vi "CRYMessages.vi"(0 "Setup in":T1={"No.VI"=0, "Category"="", "StepName"="", "Seq setup flattened"="", "Comment"="", "Steps config."=[], "Jump config"=[], "Start"=0.0, "Increment"=0.0, "Name"="Pa", "Unit"="Pa", "Y data"=1, "Y prefix"="", "Y dB ref"=1.0, "Y unit"="", "Repeat State Array"=[]} {"Repeat State Array"."Start" format="%#_5g"; "Y dB ref" format="%.1f"; "Y data" items=["dB", "Lin"]; "Start" format="%#_5g"}, 5 "Data in":T3[](array[typedef]) {"Z data" items=["dB", "Lin"]; "X data" items=["dB", "Lin"]; "Y data" items=["dB", "Lin"]; "Z dB ref" format="%.1f"; "Z axis" items=["Log", "Lin"]; "X dB ref" format="%.1f"; "X axis" items=["Log", "Lin"]; "Y axis" items=["Log", "Lin"]; "Y dB ref" format="%.1f"; "Curve"."z" format="%.2f"; "Curve"."y" format="%.2f"; "Curve"."x" format="%.2f"}, 7 "Results in":T4 {"Margin" format="%.2f"}, 9 "Seq Setup in":string, 11 "Step name":string, 12 "Hardware in":string, 13 "Calibration in":string) -> (3 "Types Out":string[](array[string]), 4 "Inserted Names Out":string[](array[string]), 6 "Data Out":T3[](array[typedef]) {"Z data" items=["dB", "Lin"]; "X data" items=["dB", "Lin"]; "Y data" items=["dB", "Lin"]; "Z dB ref" format="%.1f"; "Z axis" items=["Log", "Lin"]; "X dB ref" format="%.1f"; "X axis" items=["Log", "Lin"]; "Y axis" items=["Log", "Lin"]; "Y dB ref" format="%.1f"; "Curve"."z" format="%.2f"; "Curve"."y" format="%.2f"; "Curve"."x" format="%.2f"}, 8 "Results out":T4 {"Margin" format="%.2f"}, 10 "Wave out":T2[](array[typedef]) {"Y dB ref" format="%.1f"; "Y axis" items=["Log", "Lin"]; "Y data" items=["dB", "Lin"]; "X data" items=["dB", "Lin"]})   [LabVIEW 2013]
uses:
  Typedef Control/CRYData Cluster.ctl
  Typedef Control/CRYResult Cluster Array.ctl
  Typedef Control/CRYResult Cluster.ctl
  Typedef Control/CRYWaveform Cluster.ctl
  Typedef Control/CRYStep.ctl
  <vilib>/Utility/miscctls.llb/LVKeyNavTypeDef.ctl
  <vilib>/event_ctls.llb/eventvkey.ctl
  Program/CRYRef nums global.vi
  Task Sequence/CRYProject Run Control Global.vi
  CRYStepSetup/CRYStepSetup Global.vi
  CRYMainGlobal.vi
  SubVI/CRYMessage Global.vi
panel:
  out "Command":string
  in  "No":bool
  out "unit":string="(und)"
  in  "Numeric":dbl format="%#.5p"
  in  "Yes":bool
  in  "OK":bool
  out "serial line state":bool
  out "pattern":string
  out "Pattern read":T6={"0"=TRUE, "1"=TRUE, "2"=TRUE, "3"=TRUE, "4"=TRUE, "5"=TRUE, "6"=TRUE, "7"=TRUE}
  out "Write Pattern":T6={"0"=TRUE, "1"=TRUE, "2"=TRUE, "3"=TRUE, "4"=TRUE, "5"=TRUE, "6"=TRUE, "7"=TRUE}
  out "Time":u32(slide)=16203 caption="等待" scale=-1.0..1000.0
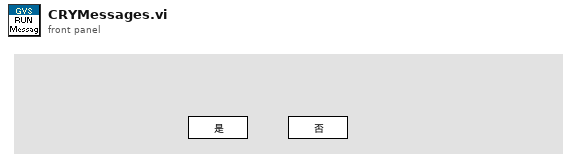
[diagram p1: front panel]
types:
  T1 = typedef "CRYStep.ctl" = cluster{"No.VI":i32, "Category":string, "StepName":string, "Seq setup flattened":string, "Comment":string, "Steps config.":bool[], "Jump config":i32[], "Start":dbl, "Increment":dbl, "Name":string, "Unit":string, "Y data":u16, "Y prefix":string, "Y dB ref":dbl, "Y unit":string, "Repeat State Array":cluster{"Start":dbl, "Increment":dbl, "Count":i32, "Num":i32}[]}
  T2 = typedef "CRYWaveform Cluster.ctl" = cluster{"Waveform":cluster{"X0":dbl, "dX":dbl, "Y":sgl[]}, "X data":u16, "Y data":u16, "Y axis":u16, "X unit":string, "Y unit":string, "Y dB ref":dbl, "display Y":bool, "display X":bool, "Overload?":bool, "Test Info":string, "Step No.":i32, "Name":string, "protected":bool, "Sqc history":string[], "Signal Channel ID":i32, "Plot Settings":cluster{"Color":u32, "Interpolation":u8, "Point Style":u8, "Line Style":u8, "Point Color":u32, "Line Width":u8, "Bar Plot Style":u8, "Fill To":i16}, "AutoProtect":bool}
  T3 = typedef "CRYData Cluster.ctl" = cluster{"Name":string, "Curve":cluster{"x":dbl, "y":dbl, "z":dbl}[], "X data":u16, "Y data":u16, "Z data":u16, "X axis":u16, "Y axis":u16, "Z axis":u16, "X unit":string, "Y unit":string, "Z unit":string, "X dB ref":dbl, "Y dB ref":dbl, "Z dB ref":dbl, "single val":bool, "protected":bool, "display X":bool, "display Y":bool, "display Z":bool, "Test Info":string, "Step No.":i32, "Plot Settings":cluster{"Color":u32, "Interpolation":u8, "Point Style":u8, "Line Style":u8, "Point Color":u32, "Line Width":u8, "Bar Plot Style":u8, "Fill To":i16}, "AutoProtect":bool}
  T4 = typedef "CRYResult Cluster Array.ctl" = T5[]
  T5 = typedef "CRYResult Cluster.ctl" = cluster{"Name":string, "Margin":dbl, "unit":string, "Verdict":bool, "Limit":string, "Max/Min":string, "protected":bool, "Step No.":i32, "Test Info":string, "AutoProtect":bool}
  T6 = cluster{"0":bool, "1":bool, "2":bool, "3":bool, "4":bool, "5":bool, "6":bool, "7":bool}
  T7 = typedef "LVKeyNavTypeDef.ctl" = cluster{"Control":bool, "Shift":bool, "Key":string}
  T8 = cluster{"Start":dbl, "Increment":dbl, "Count":i32, "Num":i32}[]
  T9 = typedef "CRYHardware.ctl" = cluster{"Name":string, "Analog I/O":u16, "Digital I/O":u16, "Channels":u8, "Dig Dev ID":u8, "N ports":u8, "Interface":u32, "Dig I/O Ports":cluster{"port #":i16, "width":i16, "direction":i32}[], "Interf settings":cluster{"Type":u16, "COM Port":u8, "Baud rate":u32, "Data bits":u32, "Parity":u16, "Stop bits":u16, "Flow control":u16, "Dev ID IEEE":u8}[], "N interfs":i32, "udev SNs":i16[], "udev enable":bool, "Channel Array":T10[], "Cal sequence":string, "SelectedIn":u16, "SelectedOut":u16, "SelectedTab":u16, "State":bool, "Help":string, "Advanced":bool, "In Audio Driver":u16, "Out Audio Driver":u16}
  T10 = typedef "CRYHardware Channel Info.ctl" = cluster{"ID":i32, "Name":string, "Digital":bool, "Input":bool, "Device Name":string, "Hardware Ch ID":u8, "Vmax (V)":dbl, "Latency (samples)":dbl, "Sampling Rate (Hz)":u32, "Bit Depth":u32, "Anti-aliasing Factor (%fs)":sgl, "DAQmx Channel":tag, "term config":i32, "Coupling":i32, "IEPE en":bool, "ASIOChannel Name":string, "Audio Driver":u16, "ASIOChannel Index":u8}
  T11 = cluster{"Type":u16, "COM Port":u8, "Baud rate":u32, "Data bits":u32, "Parity":u16, "Stop bits":u16, "Flow control":u16, "Dev ID IEEE":u8}[]
  T12 = typedef "CRYMessages Cluster.ctl" = cluster{"Name":string, "Type":u16, "Command Msg":string, "Flags":u16, "Dialog?":bool, "Numeric?":bool, "Wait?":bool, "Pause [ms]":i32, "pattern":u32, "Address":string, "Operation":i32, "bytes":i32, "Line selected":u32, "RS232 Func":u16, "Serial Ctrl lines":u16, "Interf #":u8, "GPIB func":u16, "GPIB cmd":u16, "GPIB rem en":bool, "GPIB term":i32, "Curves generated":string[], "Units":cluster{"unit":string, "dB ref":dbl, "axis":u16, "data":u16, "Common dB ref.":u16}, "Axis":u16, "Default Value":dbl, "Message Tilte":string, "Port #":i32, "Print Unit":string, "Text Format":cluster{"Size":u32, "Plain":bool, "Bold":bool, "Italic":bool, "Underline":bool, "Strikethrough":bool, "Color":u32, "Font":string}, "Help":string, "Tab Value":enum32{"Setting", "Help"}, "pattern 2":u32, "Line selected 2":u32, "H_Bits":cluster{"Bits":string[], "Invert":bool, "All":bool}[], "G_Bits":cluster{"Bits":string[], "Invert":bool, "All":bool}[]}
  T13 = cluster{"Type":u16, "COM Port":u8, "Baud rate":u32, "Data bits":u32, "Parity":u16, "Stop bits":u16, "Flow control":u16, "Dev ID IEEE":u8}
  T14 = enum32{"Invalid", "Default", "Floating", "Floating/Auto-Hide", "Modal"}
  T15 = typedef "eventvkey.ctl" = enum16{"ASCII", "Enter", "Return", "Shift", "Ctrl", "Alt", "Cmd", "Opt", "Caps", "NumLock", "Clear", "Break", "Up", "Down", "Left", "Right", "Insert", "Delete", "Home", "End", "PageUp", "PageDown", "Escape", "Help", "Pause", "ScrollLock", "F1", "F2", "F3", "F4", "F5", "F6", "F7", "F8", "F9", "F10", "F11", "F12", "F13", "F14", "F15", "F16", "F17", "F18", "F19", "F20", "F21", "F22", "F23", "F24", "Play", "VolumeUp", "VolumeDown", "Mute", "Two Byte Char"}
  T16 = enum16{"Sticks Top/Left", "Sticks Bottom/Right", "Proportional"}
  T17 = enum16{"OK", "Yes", "YesNo", "YesNoCancel", "ReplaceAppend"}
  T18 = cluster{"Size":u32, "Plain":bool, "Bold":bool, "Italic":bool, "Underline":bool, "Strikethrough":bool, "Color":u32, "Font":string}
  T19 = typedef "LVFontTypeDef.ctl" = cluster{"Font Name":string, "Size":u16, "Bold":bool, "Italic":bool, "Underline":bool, "Strikeout":bool, "Color":u32}
  T20 = typedef "LVRectTypeDef.ctl" = cluster{"Left":i16, "Top":i16, "Right":i16, "Bottom":i16}
  T21 = cluster{"unit":string, "dB ref":dbl, "axis":u16, "data":u16, "Common dB ref.":u16}
  T22 = cluster{"Numeric":dbl, "Numeric Entry":dbl, "Numeric Entry":dbl}
  T23 = cluster{"Numeric":dbl, "Numeric":dbl, "Numeric":dbl}
  T24 = cluster{"Numeric Entry":dbl, "Numeric Entry":dbl, "Numeric":dbl}
  T25 = cluster{"Numeric Entry":dbl, "Numeric Entry":dbl, "Numeric":dbl}[]
  T26 = cluster{"Bits":string[], "Invert":bool, "All":bool}[]
  T27 = cluster{"Boolean array[0]":bool, "Boolean array[1]":bool, "Boolean array[2]":bool, "Boolean array[3]":bool, "Boolean array[4]":bool, "Boolean array[5]":bool, "Boolean array[6]":bool, "Boolean array[7]":bool}
  T28 = cluster{"DIO Port Config":refnum<vi>, "DIO Port Write":refnum<vi>, "DIO Port Read":refnum<vi>}
  T29 = cluster{"COM port (1 = COM1, etc.)":i32, "VISA session (for class)":refnum<visa-resource-name>}[]
  T30 = cluster{"COM port (1 = COM1, etc.)":i32, "VISA session (for class)":refnum<visa-resource-name>}
  T31 = typedef "CRYData Cluster Array.ctl" = T3[]
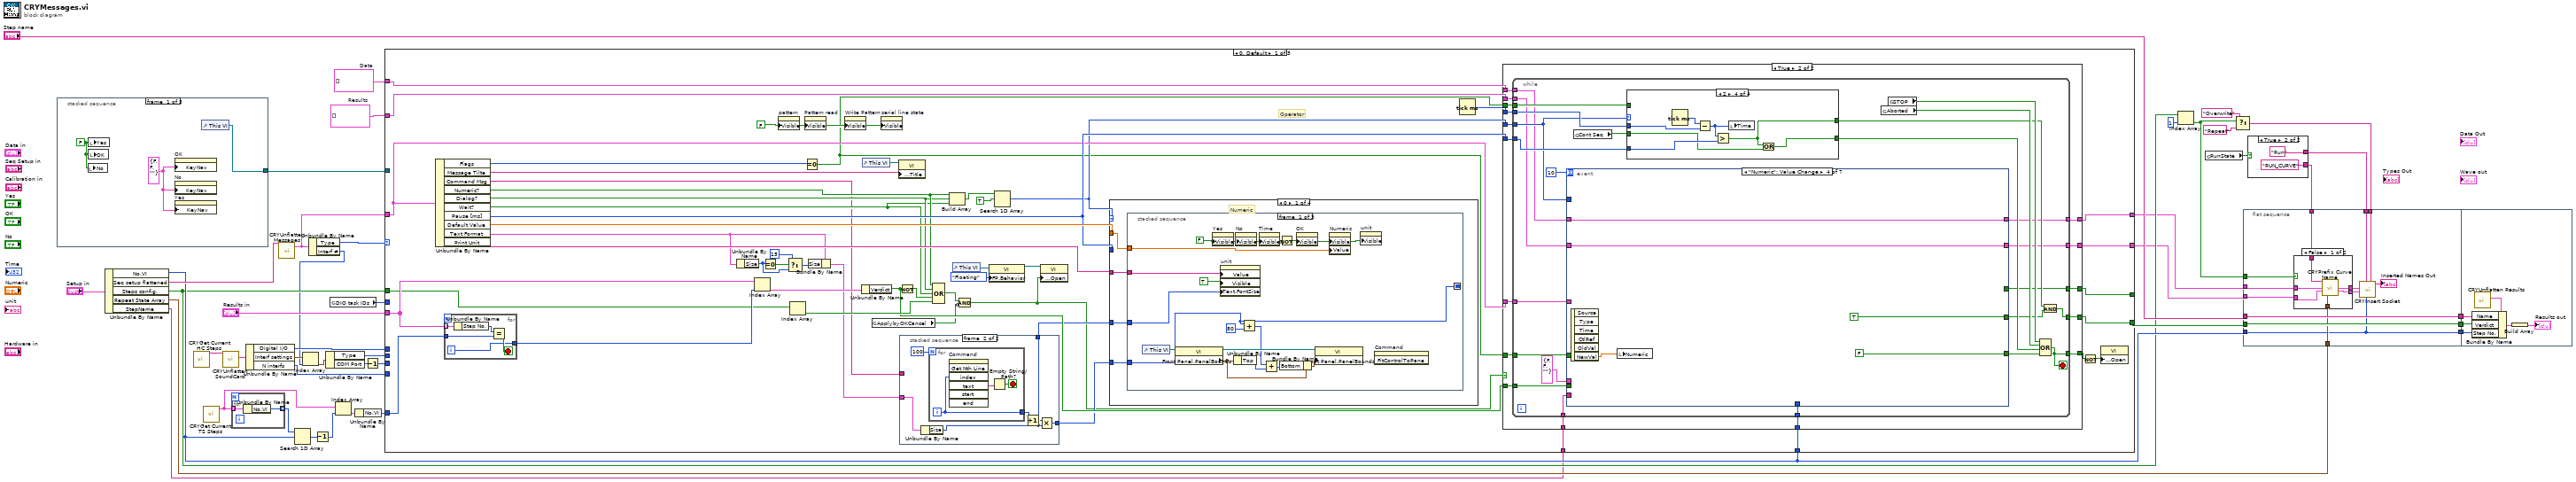
[diagram p0: block diagram]
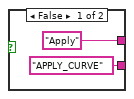
[diagram p2: hidden frame]
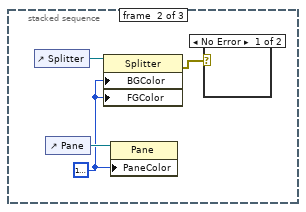
[diagram p4: hidden frame]
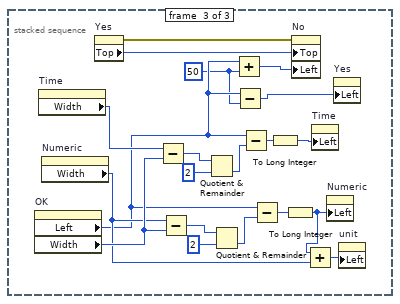
[diagram p6: hidden frame]
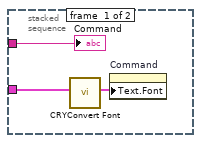
[diagram p7: hidden frame]
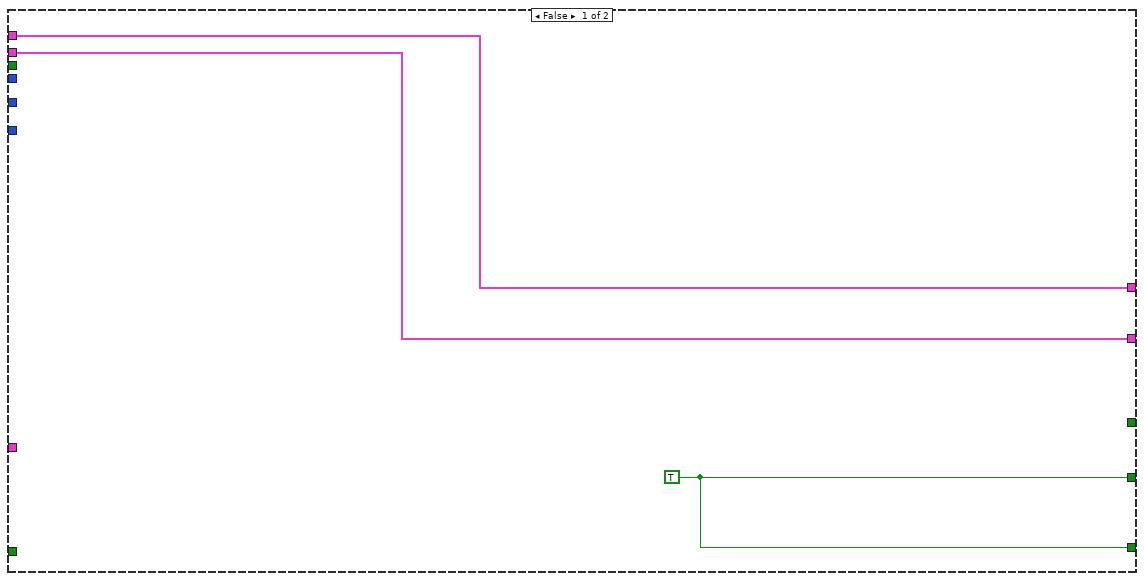
[diagram p8: hidden frame]
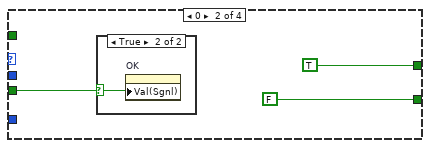
[diagram p10: hidden frame]
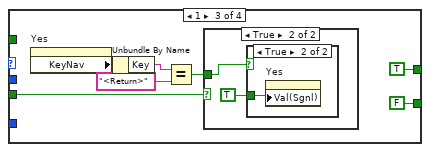
[diagram p12: hidden frame]
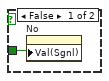
[diagram p14: hidden frame]
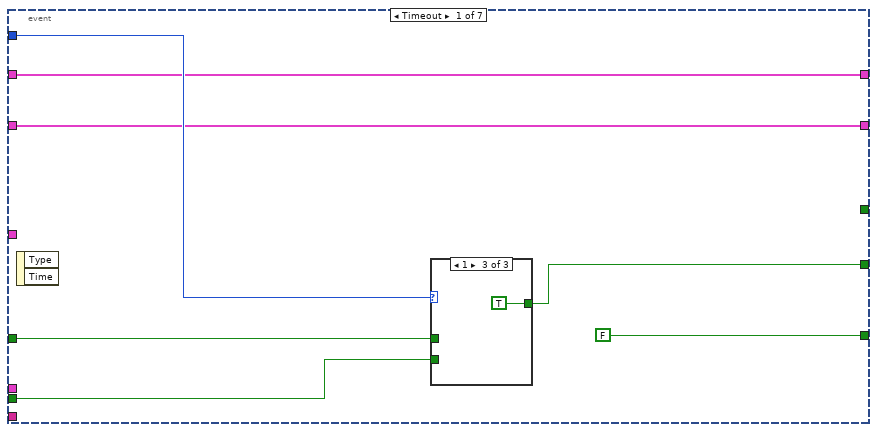
[diagram p15: hidden frame]
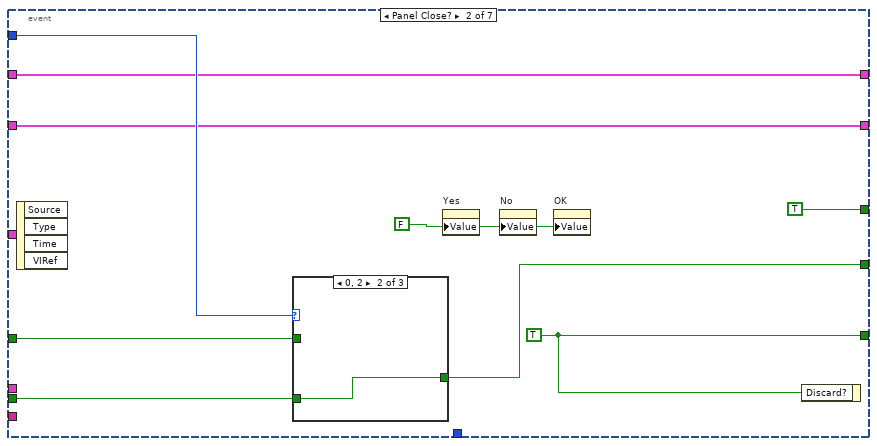
[diagram p18: hidden frame]
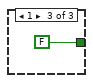
[diagram p20: hidden frame]
diagram:
  w6 = T3[] []  # Data
  w5 = T4 []  # Results
  n1 = stacked-sequence {
    tunnel: [w47 _ _] -> w29
    frame #0 {
      w45 = T7 {"Control"=FALSE, "Shift"=FALSE, "Key"=""} ("Focus Key Binding")
      w46 = FALSE ("Yes")
      n2 = local write "No"(w46) -> ()
      n3 = local write "Yes"(w46) -> ()
      n4 = local write "OK"(w46) -> ()
      n5 = property on="OK" class="Bool (strict)"("KeyNav"=w45) -> ()  [unwired: 2 in, 2 out]
      n6 = property on="No" class="Bool (strict)"("KeyNav"=w45) -> ()  [unwired: 2 in, 2 out]
      n7 = property on="Yes" class="Bool (strict)"("KeyNav"=w45) -> ()  [unwired: 2 in, 2 out]
      n8 = control-ref of="This VI"() -> (w47:refnum<vi>)
    }
    frame #1 {
      w49 = u32 16777238
      n9 = control-ref of="Splitter"() -> (w50:refnum<vi>)
      n10 = control-ref of="Pane"() -> (w51:refnum<vi>)
      n11 = property class="Splitter"(reference=w50, "BGColor"=w49, "FGColor"=w49) -> (error out=w48:errorcluster)  [unwired: 1 in, 1 out]
      n12 = property class="Pane"(reference=w51, "PaneColor"=w49) -> ()  [unwired: 1 in, 2 out]
      n13 = case shown="No Error" w48 {
        frame No Error {
        }
        frame Error {
        }
      }
    }
    frame #2 {
      w53 = 50 ("y")
      n14 = property on="OK" class="Bool (strict)"() -> ("Left"=w54:i32, "Width"=w60:u32)  [unwired: 2 in, 2 out]
      n15 = property on="Time" class="Slide (strict)"() -> ("Width"=w61:u32)  [unwired: 2 in, 2 out]
      n16 = property on="Numeric" class="DigNum (strict)"() -> ("Width"=w56:u32)  [unwired: 2 in, 2 out]
      n17 = property on="Yes" class="Bool (strict)"() -> (error out=w71:errorcluster, "Top"=w70:i32)  [unwired: 2 in, 1 out]
      n18 = Subtract(x=w61, y=w60) -> (x-y=w66:u32)
      n19 = Subtract(x=w56, y=w60) -> (x-y=w69:u32)
      n20 = Quotient & Remainder(x=w66, y=u32 2) -> (floor(x/y)=w62:u32)  [unwired: 1 out]
      n21 = Quotient & Remainder(x=w69, y=u32 2) -> (floor(x/y)=w65:u32)  [unwired: 1 out]
      n22 = Add(x=w54, y=w53) -> (x+y=w55:i32)
      n23 = Subtract(x=w54, y=w53) -> (x-y=w52:i32)
      n24 = Subtract(x=w54, y=w62) -> (x-y=w63:u32)
      n25 = Subtract(x=w54, y=w65) -> (x-y=w64:u32)
      n26 = To Long Integer(number=w63) -> (32bit integer=w59:i32)
      n27 = To Long Integer(number=w64) -> (32bit integer=w57:i32)
      n28 = property on="No" class="Bool (strict)"(error in=w71, "Top"=w70, "Left"=w55) -> ()  [unwired: 1 in, 2 out]
      n29 = Add(x=w57, y=w56) -> (x+y=w58:u32)
      n30 = property on="Time" class="Slide (strict)"("Left"=w59) -> ()  [unwired: 2 in, 2 out]
      n31 = property on="Numeric" class="DigNum (strict)"("Left"=w57) -> ()  [unwired: 2 in, 2 out]
      n32 = property on="Yes" class="Bool (strict)"("Left"=w52) -> ()  [unwired: 2 in, 2 out]
      n33 = property on="unit" class="Str"("Left"=w58) -> ()  [unwired: 2 in, 2 out]
    }
  }
  n34 = Unbundle By Name("Setup in") -> ("No.VI"=w25:i32, "Seq setup flattened"=w26:string, "Steps config."=w11:bool[], "Repeat State Array"=w12:T8, "StepName"=w2:string)
  n35 = call "CRYGet Current HC Steps.vi"() -> ("Hardware setup flattened Out"=w28:string)  [unwired: 10 in, 1 out]
  n36 = call "CRYGet Current TS Steps.vi"() -> ("Steps"=w35:T1[])  [unwired: 1 in, 10 out]
  n37 = call "CRYUnflatten SoundCard.vi"("Flatten SoundCard"=w28) -> ("SoundCard"=w30:T9)  [unwired: 10 out]
  n38 = for {
    tunnel: w35 -> [w73] mode=indexing
    tunnel: [w72] -> w34 mode=indexing
    n39 = Unbundle By Name(w73) -> ("No.VI"=w72:i32)
  }
  n40 = Unbundle By Name(w30) -> ("Digital I/O"=w21:u16, "Interf settings"=w44:T11, "N interfs"=w22:i32)
  n41 = call "CRYUnflatten Messages.vi"("Unflatten Messages"=w26) -> ("Messages"=w1:T12)  [unwired: 10 out]
  n42 = Search 1D Array(1D array=w34, element=w25) -> (index of element=w36:i32)  [unwired: 1 out]
  n43 = Unbundle By Name(w1) -> ("Type"=w41:u16, "Interf #"=w10:u8)
  n44 = Index Array(array=w44, index=w10) -> (element=w43:T13)
  n45 = Decrement(x=w36) -> (x-1=w33:i32)
  n46 = Unbundle By Name(w43) -> ("Type"=w23:u16, "COM Port"=w40:u8)
  n47 = global read "CRYRef nums global.vi" "DIO task IDs"() -> (w38:u32[])
  n48 = Index Array(array=w35, index=w33) -> (element=w37:T1)
  n49 = Unbundle By Name(w37) -> ("No.VI"=w31:i32)
  n50 = Decrement(x=w40) -> (x-1=w39:u8)
  n51 = case shown="0, Default" w41 {
    tunnel: w1 -> [w105 w458 w616]
    tunnel: w39 -> [_ _ w615]
    tunnel: w38 -> [_ w486 _]
    tunnel: [w116 w485 w614] -> w24
    tunnel: "Results in" -> [w110 _ _]
    tunnel: w31 -> [w109 _ _]
    tunnel: w29 -> [_ _ _]
    tunnel: w11 -> [w96 _ _]
    tunnel: w25 -> [w89 _ _]
    tunnel: w23 -> [_ _ w613]
    tunnel: w22 -> [_ _ w612]
    tunnel: w21 -> [_ w484 _]
    tunnel: w6 -> [w82 w482 w610]
    tunnel: w5 -> [w81 w481 w609]
    tunnel: [w80 w482 w610] -> w4
    tunnel: [w79 w481 w609] -> w3
    tunnel: w2 -> [w78 _ _]
    tunnel: [w77 _ _] -> _
    frame 0, Default {
      w118 = FALSE
      # "Operator"
      n52 = Unbundle By Name(w105) -> ("Flags"=w99:u16, "Message Tilte"=w113:string, "Command Msg"=w85:string, "Numeric?"=w103:bool, "Dialog?"=w102:bool, "Wait?"=w101:bool, "Pause [ms]"=w111:i32, "Default Value"=w119:dbl, "Text Format"=w91:T18, "Print Unit"=w106:string)
      n53 = for {
        tunnel: w110 -> [w139] mode=indexing
        tunnel: w109 -> [w137]
        tunnel: [w135] -> w108
        i -> [w135]
        stop <- w136 stop-if-true
        n54 = Unbundle By Name(w139) -> ("Step No."=w138:i32)
        n55 = Equal?(x=w138, y=w137) -> (x = y?=w136:bool)
      }
      n56 = Unbundle By Name(w91) -> ("Size"=w94:u32)
      n57 = Index Array(array=w110, index=w108) -> (element=w117:T5)
      n58 = Equal To 0?(x=w94) -> (x = 0?=w95:bool)
      n59 = property on="pattern" class="Str"("Visible"=w118) -> ()  [unwired: 2 in, 2 out]
      n60 = Select(t=u32 15, s=w95, f=w94) -> (s? t:f=w92:u32)
      n61 = Index Array(array=w96) -> (element=w107:bool)  [unwired: 1 in]
      n62 = Equal To 0?(x=w99) -> (x = 0?=w97:bool)
      n63 = property on="Pattern read" class="Clust (strict)"("Visible"=w118) -> ()  [unwired: 2 in, 2 out]
      n64 = Bundle By Name(cluster=w91, "Size"=w92) -> (w90:T18)
      n65 = property on="Write Pattern" class="Clust (strict)"("Visible"=w118) -> ()  [unwired: 2 in, 2 out]
      n66 = Unbundle By Name(w117) -> ("Verdict"=w98:bool)
      n67 = control-ref of="This VI"() -> (w120:refnum<vi>)
      n68 = global read "CRYStepSetup Global.vi" "ApplybyOKCancel"() -> (w75:bool)
      n69 = property on="serial line state" class="Bool (strict)"("Visible"=w118) -> ()  [unwired: 2 in, 2 out]
      n70 = property class="VI"(reference=w120, "Front Panel.Title"=w113) -> ()  [unwired: 1 in, 2 out]
      n71 = Not(x=w98) -> (.not. x?=w100:bool)
      n72 = stacked-sequence {
        tunnel: w90 -> [w124 w130]
        tunnel: w85 -> [w123 _]
        tunnel: [_ w128] -> w84
        tunnel: [_ w127] -> w83
        frame #0 {
          n73 = call "CRYConvert Font.vi"("Font In"=w124) -> ("Control Font"=w125:T19)  [unwired: 10 out]
          n74 = property on="Command" class="Str"("Text.Font"=w125) -> ()  [unwired: 2 in, 2 out]
          "Command" <- w123
        }
        frame #1 {
          n75 = Unbundle By Name(w130) -> ("Size"=w127:u32)
          n76 = for {
            N: 100 -> [_]
            tunnel: [w132] -> w129
            i -> [w132]
            stop <- w133 stop-if-true
            n77 = invoke on="Command" class="Str" method="Get Nth Line"("index"=w132) -> ("text"=w134:string)  [unwired: 6 in, 6 out]
            n78 = Empty String/Path?(string/path=w134) -> (empty?=w133:bool)
          }
          n79 = Increment(x=w129) -> (x+1=w126:i32)
          n80 = Multiply(x=w126, y=w127) -> (x*y=w128:u32)
        }
      }
      n81 = Compound Arithmetic op=OR(w103, w102, w101, w100, w107) -> (w76:bool)
      n82 = Build Array(w103, w102, w101) -> (w122:bool[])
      n83 = control-ref of="This VI"() -> (w88:refnum<vi>)
      n84 = Compound Arithmetic op=AND(w76, invert w75) -> (w74:bool)
      n85 = property class="VI"(reference=w88, "FP.Behavior"=T14."Floating" ("Front Panel Window:Behavior")) -> (reference out=w86:refnum<vi>)  [unwired: 1 in, 1 out]
      n86 = Search 1D Array(1D array=w122, element=TRUE) -> (index of element=w104:i32)  [unwired: 1 out]
      n87 = property class="VI"(reference=w86, "Front Panel.Open"=w74) -> ()  [unwired: 1 in, 2 out]
      n88 = case shown="0" w104 {
        tunnel: w119 -> [w352 w385 _ _]
        tunnel: w111 -> [_ _ w415 _]
        tunnel: w106 -> [w353 _ _ _]
        tunnel: w83 -> [w351 _ _ _]
        tunnel: w84 -> [w350 w384 w414 w437]
        frame 0 {
          # "Numeric"
          n89 = stacked-sequence {
            seq-local: [w355 _ _] -> [_ w376 _]
            tunnel: w353 -> [w354 _ _]
            tunnel: w352 -> [w357 _ _]
            tunnel: w351 -> [w356 _ _]
            tunnel: w350 -> [w355 _ _]
            frame #0 {
              w359 = FALSE
              n90 = control-ref of="This VI"() -> (w367:refnum<vi>)
              n91 = property class="VI"(reference=w367) -> (reference out=w364:refnum<vi>, "Front Panel.PanelBounds"=w363:T20)  [unwired: 1 in, 1 out]
              n92 = property on="Yes" class="Bool (strict)"("Visible"=w359) -> ()  [unwired: 2 in, 2 out]
              n93 = property on="unit" class="Str"("Value"=w354, "Visible"=TRUE ("Caption.Visible"), "Text.FontSize"=w356) -> ()  [unwired: 2 in, 2 out]
              n94 = Unbundle By Name(w363) -> ("Top"=w366:i16)
              n95 = property on="No" class="Bool (strict)"("Visible"=w359) -> ()  [unwired: 2 in, 2 out]
              n96 = Add(x=w355, y=i16 80) -> (x+y=w360:u32)
              n97 = property on="Time" class="Slide (strict)"("Visible"=w359) -> ()  [unwired: 2 in, 2 out]
              n98 = Add(x=w360, y=w366) -> (x+y=w365:u32)
              n99 = Not(x=w359) -> (.not. x?=w358:bool)
              n100 = Bundle By Name(cluster=w363, "Bottom"=w365) -> (w362:T20)
              n101 = property on="OK" class="Bool (strict)"("Visible"=w358) -> ()  [unwired: 2 in, 2 out]
              n102 = property class="VI"(reference=w364, "Front Panel.PanelBounds"=w362) -> ()  [unwired: 1 in, 2 out]
              n103 = property on="Numeric" class="DigNum (strict)"("Visible"=w358, "Value"=w357) -> ()  [unwired: 2 in, 2 out]
              n104 = property on="unit" class="Str"("Visible"=w358) -> ()  [unwired: 2 in, 2 out]
              n105 = invoke on="Command" class="Str" method="FitControlToPane"() -> ()  [unwired: 3 in, 3 out]
            }
            frame #1 {
              w374 = i16 35 ("x")
              n106 = control-ref of="Splitter"() -> (w382:refnum<vi>)
              n107 = Add(x=i16 10, y=w376) -> (x+y=w378:u32)
              n108 = property on="OK" class="Bool (strict)"("Value"=FALSE ("OK"), "KeyNav"=T7 {"Control"=FALSE, "Shift"=FALSE, "Key"="<Return>"} ("Focus Key Binding")) -> ()  [unwired: 2 in, 2 out]
              n109 = property class="Splitter"(reference=w382, "Position"=w378) -> (reference out=w381:refnum<vi>)  [unwired: 1 in, 1 out]
              n110 = property class="Splitter"(reference=w381, "Sizing"=T16."Sticks Top/Left", "Locked"=TRUE ("Splitter Position Locked")) -> (error out=w377:errorcluster)  [unwired: 1 in, 1 out]
              n111 = Add(x=w374, y=i16 3) -> (x+y=w373:i16)
              n112 = property on="Numeric" class="DigNum (strict)"("Top"=w373) -> ()  [unwired: 2 in, 2 out]
              n113 = property on="unit" class="Str"("Top"=w374) -> ()  [unwired: 2 in, 2 out]
              n114 = case shown="No Error" w377 {
                frame No Error {
                }
                frame Error {
                }
              }
              n115 = property on="OK" class="Bool (strict)"("Top"=70 ("Position:Top")) -> ()  [unwired: 2 in, 2 out]
            }
            frame #2 {
              n116 = property on="Numeric" class="DigNum (strict)"("Key Focus"=TRUE) -> ()  [unwired: 2 in, 2 out]
            }
          }
        }
        frame 1 {
          # "Dialog"
          n117 = stacked-sequence {
            seq-local: [w392 _] -> [_ w408]
            tunnel: w385 -> [w386 _]
            tunnel: w384 -> [w392 _]
            frame #0 {
              w390 = FALSE
              n118 = To Byte Integer(number=w386) -> (8bit integer=w389:i8)
              n119 = property on="unit" class="Str"("Visible"=w390) -> ()  [unwired: 2 in, 2 out]
              n120 = case shown="0, Default" w389 {
                tunnel: T7 {"Control"=FALSE, "Shift"=FALSE, "Key"="<Return>"} ("Focus Key Binding") -> [w402 w404]
                tunnel: T7 {"Control"=FALSE, "Shift"=FALSE, "Key"=""} ("Focus Key Binding") -> [w401 w403]
                frame 0, Default {
                  n121 = property on="No" class="Bool (strict)"("KeyNav"=w402) -> ()  [unwired: 2 in, 2 out]
                  n122 = property on="Yes" class="Bool (strict)"("KeyNav"=w401) -> ()  [unwired: 2 in, 2 out]
                }
                frame 1 {
                  n123 = property on="No" class="Bool (strict)"("KeyNav"=w403) -> ()  [unwired: 2 in, 2 out]
                  n124 = property on="Yes" class="Bool (strict)"("KeyNav"=w404) -> ()  [unwired: 2 in, 2 out]
                }
              }
              n125 = property on="OK" class="Bool (strict)"("Visible"=w390) -> ()  [unwired: 2 in, 2 out]
              n126 = property on="Numeric" class="DigNum (strict)"("Visible"=w390) -> ()  [unwired: 2 in, 2 out]
              n127 = property on="Time" class="Slide (strict)"("Visible"=w390) -> ()  [unwired: 2 in, 2 out]
              n128 = control-ref of="This VI"() -> (w400:refnum<vi>)
              n129 = Not(x=w390) -> (.not. x?=w391:bool)
              n130 = property on="Yes" class="Bool (strict)"("Visible"=w391) -> ()  [unwired: 2 in, 2 out]
              n131 = property class="VI"(reference=w400) -> (reference out=w397:refnum<vi>, "Front Panel.PanelBounds"=w396:T20)  [unwired: 1 in, 1 out]
              n132 = property on="No" class="Bool (strict)"("Visible"=w391) -> ()  [unwired: 2 in, 2 out]
              n133 = Unbundle By Name(w396) -> ("Top"=w399:i16)
              n134 = Add(x=w392, y=i16 60) -> (x+y=w393:u32)
              n135 = Add(x=w393, y=w399) -> (x+y=w398:u32)
              n136 = Bundle By Name(cluster=w396, "Bottom"=w398) -> (w395:T20)
              n137 = property class="VI"(reference=w397, "Front Panel.PanelBounds"=w395) -> ()  [unwired: 1 in, 2 out]
            }
            frame #1 {
              w407 = i16 40 ("x")
              n138 = control-ref of="Splitter"() -> (w413:refnum<vi>)
              n139 = Add(x=i16 10, y=w408) -> (x+y=w409:u32)
              n140 = invoke on="Command" class="Str" method="FitControlToPane"() -> ()  [unwired: 3 in, 3 out]
              n141 = property class="Splitter"(reference=w413, "Position"=w409) -> (reference out=w412:refnum<vi>)  [unwired: 1 in, 1 out]
              n142 = property class="Splitter"(reference=w412, "Sizing"=T16."Sticks Top/Left", "Locked"=TRUE ("Splitter Position Locked")) -> (error out=w406:errorcluster)  [unwired: 1 in, 1 out]
              n143 = property on="Yes" class="Bool (strict)"("Top"=w407) -> ()  [unwired: 2 in, 2 out]
              n144 = property on="No" class="Bool (strict)"("Top"=w407) -> ()  [unwired: 2 in, 2 out]
              n145 = case shown="No Error" w406 {
                frame No Error {
                }
                frame Error {
                }
              }
            }
          }
        }
        frame 2 {
          # "Wait"
          n146 = stacked-sequence {
            seq-local: [w416 _] -> [_ w431]
            tunnel: w415 -> [w427 _]
            tunnel: w414 -> [w416 _]
            frame #0 {
              w417 = FALSE
              n147 = control-ref of="This VI"() -> (w425:refnum<vi>)
              n148 = property on="Time" class="Slide (strict)"("标尺.范围:最大值"=w427) -> ()  [unwired: 2 in, 2 out]
              n149 = property class="VI"(reference=w425) -> (reference out=w422:refnum<vi>, "Front Panel.PanelBounds"=w421:T20)  [unwired: 1 in, 1 out]
              n150 = property on="unit" class="Str"("Visible"=w417) -> ()  [unwired: 2 in, 2 out]
              n151 = property on="OK" class="Bool (strict)"("Visible"=w417) -> ()  [unwired: 2 in, 2 out]
              n152 = Add(x=w416, y=i16 60) -> (x+y=w418:u32)
              n153 = property on="Numeric" class="DigNum (strict)"("Visible"=w417) -> ()  [unwired: 2 in, 2 out]
              n154 = Unbundle By Name(w421) -> ("Top"=w424:i16)
              n155 = property on="Yes" class="Bool (strict)"("Visible"=w417) -> ()  [unwired: 2 in, 2 out]
              n156 = Add(x=w418, y=w424) -> (x+y=w423:u32)
              n157 = property on="No" class="Bool (strict)"("Visible"=w417) -> ()  [unwired: 2 in, 2 out]
              n158 = Bundle By Name(cluster=w421, "Bottom"=w423) -> (w420:T20)
              n159 = Not(x=w417) -> (.not. x?=w426:bool)
              n160 = property on="Time" class="Slide (strict)"("Visible"=w426) -> ()  [unwired: 2 in, 2 out]
              n161 = property class="VI"(reference=w422, "Front Panel.PanelBounds"=w420) -> ()  [unwired: 1 in, 2 out]
            }
            frame #1 {
              n162 = control-ref of="Splitter"() -> (w436:refnum<vi>)
              n163 = invoke on="Command" class="Str" method="FitControlToPane"() -> ()  [unwired: 3 in, 3 out]
              n164 = Add(x=i16 10, y=w431) -> (x+y=w432:u32)
              n165 = property class="Splitter"(reference=w436, "Position"=w432) -> (reference out=w435:refnum<vi>)  [unwired: 1 in, 1 out]
              n166 = property class="Splitter"(reference=w435, "Sizing"=T16."Sticks Top/Left", "Locked"=TRUE ("Splitter Position Locked")) -> (error out=w429:errorcluster)  [unwired: 1 in, 1 out]
              n167 = property on="Time" class="Slide (strict)"("Top"=i16 40 ("x")) -> ()  [unwired: 2 in, 2 out]
              n168 = case shown="No Error" w429 {
                frame No Error {
                }
                frame Error {
                }
              }
            }
          }
        }
        frame Default {
          # "Nothing"
          n169 = stacked-sequence {
            seq-local: [w438 _] -> [_ w451]
            tunnel: w437 -> [w438 _]
            frame #0 {
              w439 = FALSE
              n170 = control-ref of="This VI"() -> (w447:refnum<vi>)
              n171 = property class="VI"(reference=w447) -> (reference out=w444:refnum<vi>, "Front Panel.PanelBounds"=w443:T20)  [unwired: 1 in, 1 out]
              n172 = property on="unit" class="Str"("Visible"=w439) -> ()  [unwired: 2 in, 2 out]
              n173 = property on="OK" class="Bool (strict)"("Visible"=w439) -> ()  [unwired: 2 in, 2 out]
              n174 = Unbundle By Name(w443) -> ("Top"=w446:i16)
              n175 = property on="Numeric" class="DigNum (strict)"("Visible"=w439) -> ()  [unwired: 2 in, 2 out]
              n176 = Add(x=w438, y=i16 30) -> (x+y=w440:u32)
              n177 = property on="Yes" class="Bool (strict)"("Visible"=w439) -> ()  [unwired: 2 in, 2 out]
              n178 = Add(x=w440, y=w446) -> (x+y=w445:u32)
              n179 = property on="No" class="Bool (strict)"("Visible"=w439) -> ()  [unwired: 2 in, 2 out]
              n180 = Bundle By Name(cluster=w443, "Bottom"=w445) -> (w442:T20)
              n181 = property on="Time" class="Slide (strict)"("Visible"=w439) -> ()  [unwired: 2 in, 2 out]
              n182 = property class="VI"(reference=w444, "Front Panel.PanelBounds"=w442) -> ()  [unwired: 1 in, 2 out]
            }
            frame #1 {
              n183 = control-ref of="Splitter"() -> (w456:refnum<vi>)
              n184 = Add(x=i16 10, y=w451) -> (x+y=w452:u32)
              n185 = property class="Splitter"(reference=w456, "Position"=w452) -> (reference out=w455:refnum<vi>, error out=w450:errorcluster)  [unwired: 1 in]
              n186 = invoke on="Command" class="Str" method="FitControlToPane"() -> ()  [unwired: 3 in, 3 out]
              n187 = property class="Splitter"(reference=w455, error in=w450, "Sizing"=T16."Sticks Top/Left", "Locked"=TRUE ("Splitter Position Locked")) -> (error out=w449:errorcluster)  [unwired: 1 out]
              n188 = case shown="No Error" w449 {
                frame No Error {
                }
                frame Error {
                }
              }
            }
          }
        }
      }
      n189 = Tick Count (ms)() -> (millisecond timer value=w112:u32)
      n190 = case shown="True" w74 {
        tunnel: [w142 w156] -> w116
        tunnel: [w142 w158] -> w114
        tunnel: w104 -> [_ w157]
        tunnel: w98 -> [_ w153]
        tunnel: w112 -> [_ w155]
        tunnel: w111 -> [_ w154]
        tunnel: w105 -> [_ w152]
        tunnel: w97 -> [_ w151]
        tunnel: w97 -> [_ w150]
        tunnel: w89 -> [_ w149]
        tunnel: w82 -> [w141 w148]
        tunnel: w81 -> [w140 w147]
        tunnel: [w141 w146] -> w80
        tunnel: [w140 w145] -> w79
        tunnel: w78 -> [_ w144]
        tunnel: [_ w143] -> w77
        frame False {
          w142 = TRUE
        }
        frame True {
          n191 = while {
            tunnel: [w180] -> w158
            tunnel: w157 -> [w178]
            tunnel: [w168] -> w156
            tunnel: w155 -> [w182]
            tunnel: w154 -> [w181]
            tunnel: w153 -> [w177]
            tunnel: w152 -> [w175]
            tunnel: w151 -> [w171]
            tunnel: w150 -> [w167]
            tunnel: w149 -> [w165]
            tunnel: w148 -> [w164]
            tunnel: w147 -> [w163]
            tunnel: [w162] -> w146
            tunnel: [w161] -> w145
            tunnel: w144 -> [w160]
            tunnel: [w159] -> w143
            stop <- w180 stop-if-true
            n192 = event shown="[3] \"Numeric\": Value Change" {
              selector: _ -> [_ _ _ _ _ _ _]
              dyn-events: _ -> [_ _ _ _ _ _ _]
              timeout: 10 -> [_ _ _ _ _ _ _]
              tunnel: [w211 w223 w233 TRUE ("NewVal") w309 w320 w329] -> w170
              tunnel: [FALSE w222 w233 FALSE ("NewVal") w304 w316 w331] -> w172
              tunnel: w178 -> [w213 w225 _ _ _ _ w332]
              tunnel: w177 -> [w212 w224 _ _ _ _ _]
              tunnel: w175 -> [_ _ w243 _ _ _ _]
              tunnel: w171 -> [w210 w221 _ _ _ _ w330]
              tunnel: T7 {"Control"=FALSE, "Shift"=FALSE, "Key"=""} ("Focus Key Binding") -> [_ _ w235 _ w303 w315 _]
              tunnel: w165 -> [_ _ w234 _ w302 w314 _]
              tunnel: w164 -> [w209 w220 _ w294 w299 w311 w323]
              tunnel: w163 -> [w208 w219 w232 w293 _ _ w322]
              tunnel: [w209 w220 w230 w294 w299 w311 w323] -> w162
              tunnel: [w208 w219 w232 w293 w300 w312 w322] -> w161
              tunnel: w160 -> [_ _ w231 _ w298 w310 _]
              tunnel: [_ TRUE _ _ _ _ _] -> w159
              event Timeout {
                n193 = event-data() -> ()  [unwired: 3 out]
                n194 = case shown="1" w213 {
                  tunnel: w212 -> [_ w216 _]
                  tunnel: [w215 w216 TRUE ("NewVal")] -> w211
                  tunnel: w210 -> [w215 _ _]
                  frame Default {
                  }
                  frame 0, 2 {
                  }
                  frame 1 {
                  }
                }
              }
              event Panel Close? {
                w226 = FALSE ("OK")
                w222 = TRUE
                n195 = event-data() -> ()  [unwired: 5 out]
                n196 = case shown="0, 2" w225 {
                  tunnel: w224 -> [_ w228 _]
                  tunnel: [w227 w228 FALSE ("NewVal")] -> w223
                  tunnel: w221 -> [w227 _ _]
                  frame Default {
                  }
                  frame 0, 2 {
                  }
                  frame 1 {
                  }
                }
                n197 = property on="Yes" class="Bool (strict)"("Value"=w226) -> ()  [unwired: 2 in, 2 out]
                n198 = property on="No" class="Bool (strict)"("Value"=w226) -> ()  [unwired: 2 in, 2 out]
                n199 = property on="OK" class="Bool (strict)"("Value"=w226) -> ()  [unwired: 2 in, 2 out]
                n200 = event-data("Discard?"=w222) -> ()  [unwired: 1 in, 1 out]
              }
              event "OK": Value Change {
                w233 = TRUE ("NewVal")
                w245 = u16 1 ("Z axis")
                n201 = event-data() -> ("CtlRef"=w237:refnum<vi>)  [unwired: 6 out]
                n202 = property class="Bool (strict)"(reference=w237, "Value"=FALSE, "KeyNav"=w235) -> ()  [unwired: 1 in, 2 out]
                n203 = Unbundle By Name(w243) -> ("Units"=w242:T21, "Print Unit"=w241:string, "Axis"=w240:u16)
                n204 = local read "Numeric"() -> (w246:dbl)
                n205 = Unbundle By Name(w242) -> ("dB ref"=w239:dbl, "axis"=w244:u16)
                n206 = call "CRYUnflatten Data.vi"() -> ("Datum"=w250:T3)  [unwired: 1 in, 10 out]
                n207 = case shown="2" w240 {
                  tunnel: [w264 w278 w292] -> w249
                  tunnel: w246 -> [w262 w274 w287]
                  tunnel: w250 -> [w261 w277 w291]
                  tunnel: [w260 w276 w290] -> w251
                  tunnel: w241 -> [w259 w275 w289]
                  tunnel: w244 -> [w253 w269 w281]
                  tunnel: w239 -> [w252 w265 w279]
                  frame 0, Default {
                    w256 = u16 1 ("Y data")
                    w257 = FALSE ("display Y")
                    w263 = 0.0 ("Numeric Entry")
                    # "x"
                    n208 = Bundle By Name(cluster=w261, "Y unit"="", "Z unit"="deg.", "X data"=w253, "Y data"=w256, "Z data"=w256, "X axis"=w256, "X unit"=w259, "display X"=TRUE, "display Y"=w257, "display Z"=w257, "X dB ref"=w252) -> (w260:T3)
                    n209 = Bundle("Numeric"=w262, "Numeric Entry"=w263, "Numeric Entry"=w263) -> (w264:T22)  [unwired: 1 out]
                  }
                  frame 1 {
                    w266 = 0.0 ("Numeric")
                    w268 = u16 1 ("X data")
                    w273 = FALSE ("display X")
                    # "y"
                    n210 = Bundle("Numeric"=w266, "Numeric"=w274, "Numeric"=w266) -> (w278:T23)  [unwired: 1 out]
                    n211 = Bundle By Name(cluster=w277, "X data"=w268, "Y data"=w269, "Z data"=w268, "X axis"=u16 0, "Z unit"="deg.", "X unit"="Hz", "Y unit"=w275, "display X"=w273, "display Y"=TRUE, "display Z"=w273, "Y dB ref"=w265) -> (w276:T3)
                  }
                  frame 2 {
                    w280 = u16 1 ("X data")
                    w286 = FALSE ("display X")
                    w288 = 0.0 ("Numeric Entry")
                    # "z"
                    n212 = Bundle("Numeric Entry"=w288, "Numeric Entry"=w288, "Numeric"=w287) -> (w292:T24)  [unwired: 1 out]
                    n213 = Bundle By Name(cluster=w291, "X data"=w280, "Y data"=w280, "Z data"=w281, "X axis"=u16 0, "X unit"="Hz", "Y unit"="", "Z unit"=w289, "display X"=w286, "display Y"=w286, "display Z"=TRUE, "Z dB ref"=w279) -> (w290:T3)
                  }
                }
                n214 = Build Array(w249) -> (w247:T25)
                n215 = Bundle By Name(cluster=w251, "Z axis"=w245, "Y axis"=w245, "Name"=w231, "single val"=TRUE ("Bundle Element"), "Curve"=w247, "Step No."=w234) -> (w238:T3)
                n216 = Build Array(w238) -> (w230:T3[])
              }
              event "Numeric": Value Change {
                n217 = event-data() -> ("NewVal"=w297:dbl)  [unwired: 6 out]
                n218 = local write "Numeric"(w297) -> ()
              }
              event "Yes": Value Change {
                w309 = TRUE ("NewVal")
                n219 = event-data() -> ("CtlRef"=w306:refnum<vi>, "NewVal"=w304:bool)  [unwired: 5 out]
                n220 = property class="Bool (strict)"(reference=w306, "Value"=FALSE, "KeyNav"=w303) -> ()  [unwired: 1 in, 2 out]
                n221 = call "CRYUnflatten Results.vi"() -> ("Result"=w301:T5)  [unwired: 9 in, 2 out]
                n222 = Bundle By Name(cluster=w301, "Name"=w298, "Verdict"=w309, "Step No."=w302, "Margin"=1.0) -> (w307:T5)
                n223 = Build Array(w307) -> (w300:T5[])
              }
              event "No": Value Change {
                w320 = FALSE ("NewVal")
                n224 = event-data() -> ("CtlRef"=w318:refnum<vi>, "NewVal"=w316:bool)  [unwired: 5 out]
                n225 = property class="Bool (strict)"(reference=w318, "Value"=FALSE, "KeyNav"=w315) -> ()  [unwired: 1 in, 2 out]
                n226 = call "CRYUnflatten Results.vi"() -> ("Result"=w313:T5)  [unwired: 9 in, 2 out]
                n227 = Bundle By Name(cluster=w313, "Name"=w310, "Verdict"=w320, "Step No."=w314, "Margin"=0.0) -> (w319:T5)
                n228 = Build Array(w319) -> (w312:T5[])
              }
              event Key Down {
                n229 = event-data() -> ("VKey"=w327:T15)  [unwired: 10 out]
                n230 = Equal?(x=w327, y=eventvkey."Return") -> (x = y?=w325:bool)
                n231 = Equal?(x=w327, y=eventvkey."Enter") -> (x = y?=w326:bool)
                n232 = Or(x=w326, y=w325) -> (x .or. y?=w324:bool)
                n233 = case shown="True" w324 {
                  tunnel: w332 -> [_ w337]
                  tunnel: [_ w336] -> w331
                  tunnel: w330 -> [_ w335]
                  tunnel: [_ w334] -> w329
                  frame False {
                  }
                  frame True {
                    n234 = case shown="1" w337 {
                      tunnel: [TRUE FALSE ("Cont Seq") FALSE ("Cont Seq") _] -> w336
                      tunnel: w335 -> [w338 _ _ _]
                      tunnel: [w338 _ _ _] -> w334
                      frame Default {
                      }
                      frame 0 {
                        n235 = property on="OK" class="Bool (strict)"("Val(Sgnl)"=TRUE ("Value (Signaling)")) -> ()  [unwired: 2 in, 2 out]
                      }
                      frame 1 {
                        n236 = property on="Yes" class="Bool (strict)"() -> ("KeyNav"=w347:T7)  [unwired: 2 in, 2 out]
                        n237 = Unbundle By Name(w347) -> ("Key"=w343:string)
                        n238 = Equal?(x=w343, y="<Return>") -> (x = y?=w342:bool)
                        n239 = case shown="True" w342 {
                          tunnel: TRUE ("Cont Seq") -> [w348 w349]
                          frame False {
                            n240 = property on="No" class="Bool (strict)"("Val(Sgnl)"=w348) -> ()  [unwired: 2 in, 2 out]
                          }
                          frame True {
                            n241 = property on="Yes" class="Bool (strict)"("Val(Sgnl)"=w349) -> ()  [unwired: 2 in, 2 out]
                          }
                        }
                      }
                      frame 2 {
                      }
                    }
                  }
                }
              }
            }
            n242 = global read "CRYProject Run Control Global.vi" "Cont Seq"() -> (w173:bool)
            n243 = case shown="2" w178 {
              tunnel: w182 -> [_ _ _ w206]
              tunnel: w181 -> [_ _ _ w205]
              tunnel: [w185 FALSE ("Cont Seq") FALSE ("Cont Seq") w202] -> w179
              tunnel: w173 -> [w185 w188 w196 w203]
              tunnel: [w184 TRUE TRUE w201] -> w169
              tunnel: w167 -> [w184 _ _ _]
              frame Default {
              }
              frame 0 {
                n244 = case shown="True" w188 {
                  selector: w188 -> [_ w189]
                  frame False {
                  }
                  frame True {
                    n245 = property on="OK" class="Bool (strict)"("Val(Sgnl)"=w189) -> ()  [unwired: 2 in, 2 out]
                  }
                }
              }
              frame 1 {
                n246 = property on="Yes" class="Bool (strict)"() -> ("KeyNav"=w193:T7)  [unwired: 2 in, 2 out]
                n247 = Unbundle By Name(w193) -> ("Key"=w194:string)
                n248 = Equal?(x=w194, y="<Return>") -> (x = y?=w192:bool)
                n249 = case shown="True" w196 {
                  tunnel: w192 -> [_ w198]
                  frame False {
                  }
                  frame True {
                    n250 = case shown="True" w198 {
                      tunnel: TRUE ("Cont Seq") -> [w199 w200]
                      frame False {
                        n251 = property on="No" class="Bool (strict)"("Val(Sgnl)"=w199) -> ()  [unwired: 2 in, 2 out]
                      }
                      frame True {
                        n252 = property on="Yes" class="Bool (strict)"("Val(Sgnl)"=w200) -> ()  [unwired: 2 in, 2 out]
                      }
                    }
                  }
                }
              }
              frame 2 {
                n253 = Tick Count (ms)() -> (millisecond timer value=w207:u32)
                n254 = Subtract(x=w207, y=w206) -> (x-y=w204:u32)
                n255 = Greater?(x=w204, y=w205) -> (0:w201:bool)
                n256 = local write "Time"(w204) -> ()
                n257 = Or(x=w201, y=w203) -> (x .or. y?=w202:bool)
              }
            }
            n258 = global read "CRYProject Run Control Global.vi" "Aborted"() -> (w174:bool)
            n259 = global read "CRYMainGlobal.vi" "STOP"() -> (w176:bool)
            n260 = Compound Arithmetic op=OR(w176, w174, w179, w172) -> (w180:bool)
            n261 = And(x=w169, y=w170) -> (x .and. y?=w168:bool)
          }
        }
      }
      n262 = Not(x=w114) -> (.not. x?=w115:bool)
      n263 = property class="VI"("Front Panel.Open"=w115) -> ()  [unwired: 2 in, 2 out]
    }
    frame 1 {
      n264 = Unbundle By Name(w458) -> ("G_Bits"=w468:T26, "Line selected"=w475:u32, "pattern"=w477:u32, "Line selected 2"=w470:u32, "pattern 2"=w469:u32, "H_Bits"=w467:T26)
      n265 = Greater Than 0?(x=w484) -> (x > 0?=w483:bool)
      n266 = Number To Boolean Array(number=w477) -> (Boolean array=w478:bool[])
      n267 = Number To Boolean Array(number=w475) -> (Boolean array=w480:bool[])
      n268 = Number To Boolean Array(number=w469) -> (Boolean array=w473:bool[])
      n269 = Number To Boolean Array(number=w470) -> (Boolean array=w471:bool[])
      n270 = Array To Cluster(array=w478) -> (cluster=w476:T27)
      n271 = Array To Cluster(array=w480) -> (cluster=w479:T27)
      n272 = Array To Cluster(array=w473) -> (cluster=w474:T27)
      n273 = Array To Cluster(array=w471) -> (cluster=w472:T27)
      n274 = call "CRYDigital IO Update.vi"("Pattern"=w476, "Line selected"=w479, "Bits Cluster"=w468) -> ("Pattern Out"=w460:T6)  [unwired: 8 in]
      n275 = call "CRYDigital IO Update.vi"("Pattern"=w474, "Line selected"=w472, "Bits Cluster"=w467) -> ("Pattern Out"=w459:T6)  [unwired: 8 in]
      n276 = Cluster To Array(cluster=w459) -> (array=w464:bool[])
      n277 = Cluster To Array(cluster=w460) -> (array=w461:bool[])
      n278 = Boolean Array To Number(Boolean array=w464) -> (number=w463:u32)
      n279 = Boolean Array To Number(Boolean array=w461) -> (number=w462:u32)
      n280 = To Unsigned Long Integer(number=w463) -> (unsigned 32bit integer=w465:u32)
      n281 = To Unsigned Long Integer(number=w462) -> (unsigned 32bit integer=w466:u32)
      n282 = Bundle By Name(cluster=w458, "pattern"=w466, "pattern 2"=w465) -> (w457:T12)
      n283 = disable-structure shown="Enabled" {
        disable-tunnel: w457 -> [w490 w588]
        disable-tunnel: w486 -> [w489 _]
        disable-tunnel: [w488 w563] -> w485
        disable-tunnel: w483 -> [w487 _]
        frame Disabled {
          n284 = case shown="True" w487 {
            tunnel: w490 -> [_ w515]
            tunnel: w489 -> [_ w503]
            tunnel: [FALSE ("Verdict") w498] -> w488
            frame False {
              n285 = call "CRYGet Error Message.vi"("Error No"=1 ("No"), "Kind"="Messages") -> ("Message"=w494:string, "Window Title"=w493:string)  [unwired: 4 in, 4 out]
              n286 = call "CRYMessage Dialog.vi"("Window Title"=w493, "Message Content"=w494) -> ()  [unwired: 8 in, 2 out]
            }
            frame True {
              w497 = FALSE
              # "Digital I/O"
              n287 = Unbundle By Name(w515) -> ("Wait?"=w510:bool, "Pause [ms]"=w509:i32, "Operation"=w508:i32, "pattern"=w507:u32, "Line selected"=w506:u32, "Flags"=w505:u16, "Address"=w504:string)
              n288 = Not(x=w497) -> (.not. x?=w499:bool)
              n289 = property on="OK" class="Bool (strict)"("Visible"=w497) -> ()  [unwired: 2 in, 2 out]
              n290 = property on="Yes" class="Bool (strict)"("Visible"=w497) -> ()  [unwired: 2 in, 2 out]
              n291 = property on="pattern" class="Str"("Visible"=w499) -> ()  [unwired: 2 in, 2 out]
              n292 = property on="No" class="Bool (strict)"("Visible"=w497) -> ()  [unwired: 2 in, 2 out]
              n293 = property on="Numeric" class="DigNum (strict)"("Visible"=w497) -> ()  [unwired: 2 in, 2 out]
              n294 = global read "CRYRef nums global.vi" "DIO VI ref nums"() -> (w512:T28)
              n295 = property on="Time" class="Slide (strict)"("Visible"=w497) -> ()  [unwired: 2 in, 2 out]
              n296 = property on="unit" class="Str"("Visible"=w497) -> ()  [unwired: 2 in, 2 out]
              n297 = Decimal String To Number(string=w504) -> (number=w511:i32)  [unwired: 3 out]
              n298 = property on="serial line state" class="Bool (strict)"("Visible"=w497) -> ()  [unwired: 2 in, 2 out]
              n299 = Index Array(array=w503, index=w511) -> (element=w502:u32)
              n300 = Unbundle By Name(w512) -> ("DIO Port Write"=w514:refnum<vi>, "DIO Port Read"=w513:refnum<vi>)
              n301 = case shown="1" w508 {
                tunnel: [w534 w557] -> w498
                tunnel: [TRUE FALSE] -> w501
                tunnel: [w526 w546] -> w496
                tunnel: w509 -> [w529 w548]
                tunnel: w513 -> [_ w547]
                tunnel: w514 -> [w527 _]
                tunnel: w510 -> [w524 w545]
                tunnel: w507 -> [w521 w540]
                tunnel: w506 -> [w522 w539]
                tunnel: w505 -> [w520 _]
                tunnel: w502 -> [w523 w542]
                frame 1 {
                  # "Write"
                  n302 = call-by-ref "?"(reference=w527, "line mask"=w522, "pattern"=w521, "task ID"=w523) -> (error out=w528:errorcluster, "error out"=w530:errorcluster)  [unwired: 8 in, 2 out]
                  n303 = Unbundle By Name(w530) -> ("status"=w531:bool)
                  n304 = case shown="True" w524 {
                    tunnel: w529 -> [_ w535]
                    tunnel: w528 -> [_ _]
                    frame False {
                    }
                    frame True {
                      n305 = Wait (ms)(milliseconds to wait=w535) -> ()  [unwired: 1 out]
                    }
                  }
                  n306 = Number To Boolean Array(number=w521) -> (Boolean array=w533:bool[])
                  n307 = Array To Cluster(array=w533) -> (cluster=→"Write Pattern":T27)
                  n308 = case shown="..0" w520 {
                    tunnel: [TRUE ("Verdict") FALSE ("Verdict")] -> w534
                    frame ..0 {
                    }
                    frame 1.. {
                    }
                  }
                  n309 = Select(t=w530, s=w531, f=w528) -> (s? t:f=w526:errorcluster)
                }
                frame 0, Default {
                  # "Read"
                  n310 = case shown="True" w545 {
                    tunnel: w548 -> [_ w560]
                    tunnel: [w558 w559] -> w541
                    tunnel: w542 -> [w558 w559]
                    frame False {
                    }
                    frame True {
                      n311 = Wait (ms)(milliseconds to wait=w560) -> ()  [unwired: 1 out]
                    }
                  }
                  n312 = call-by-ref "?"(reference=w547, "task ID"=w541) -> (error out=w553:errorcluster, "error out"=w543:errorcluster, "pattern"=w550:u32)  [unwired: 9 in, 2 out]
                  n313 = Unbundle By Name(w543) -> ("status"=w554:bool)
                  n314 = And(x=w550, y=w539) -> (x .and. y?=w549:u32)
                  n315 = And(x=w540, y=w539) -> (x .and. y?=w544:u32)
                  n316 = Format Into String(format string="%08b", w550) -> (resulting string=→"pattern":string)  [unwired: 2 in, 1 out]
                  n317 = Number To Boolean Array(number=w550) -> (Boolean array=w556:bool[])
                  n318 = Select(t=w543, s=w554, f=w553) -> (s? t:f=w546:errorcluster)
                  n319 = Equal?(x=w549, y=w544) -> (x = y?=w557:bool)
                  n320 = Array To Cluster(array=w556) -> (cluster=→"Pattern read":T27)
                }
              }
              n321 = property on="Pattern read" class="Clust (strict)"("Visible"=w501) -> ()  [unwired: 2 in, 2 out]
              n322 = case shown="No Error" w496 {
                selector: w496 -> [_ w519]
                frame No Error {
                }
                frame Error {
                  n323 = Unbundle By Name(w519) -> ("source"=w516:string)
                  n324 = call "CRYGet Error Message.vi"() -> ("Window Title"=w517:string)  [unwired: 6 in, 5 out]
                  n325 = call "CRYMessage Dialog.vi"("Window Title"=w517, "YesNoCancel"=T17."OK", "Message Content"=w516) -> ()  [unwired: 7 in, 2 out]
                }
              }
              n326 = Not(x=w501) -> (.not. x?=w500:bool)
              n327 = property on="Write Pattern" class="Clust (strict)"("Visible"=w500) -> ()  [unwired: 2 in, 2 out]
            }
          }
        }
        frame Enabled {
          w589 = FALSE
          n328 = Unbundle By Name(w588) -> ("pattern"=w587:u32, "Line selected"=w586:u32, "pattern 2"=w576:u32, "Line selected 2"=w574:u32, "Flags"=w571:u16)
          n329 = Not(x=w589) -> (.not. x?=w590:bool)
          n330 = property on="OK" class="Bool (strict)"("Visible"=w589) -> ()  [unwired: 2 in, 2 out]
          n331 = property on="Yes" class="Bool (strict)"("Visible"=w589) -> ()  [unwired: 2 in, 2 out]
          n332 = property on="pattern" class="Str"("Visible"=w590) -> ()  [unwired: 2 in, 2 out]
          n333 = property on="No" class="Bool (strict)"("Visible"=w589) -> ()  [unwired: 2 in, 2 out]
          n334 = property on="Numeric" class="DigNum (strict)"("Visible"=w589) -> ()  [unwired: 2 in, 2 out]
          n335 = property on="Time" class="Slide (strict)"("Visible"=w589) -> ()  [unwired: 2 in, 2 out]
          n336 = property on="unit" class="Str"("Visible"=w589) -> ()  [unwired: 2 in, 2 out]
          n337 = To Unsigned Byte Integer(number=w587) -> (unsigned 8bit integer=w583:u8)
          n338 = To Unsigned Byte Integer(number=w586) -> (unsigned 8bit integer=w582:u8)
          n339 = To Unsigned Byte Integer(number=w576) -> (unsigned 8bit integer=w573:u8)
          n340 = To Unsigned Byte Integer(number=w574) -> (unsigned 8bit integer=w572:u8)
          n341 = global read "CRYMessage Global.vi" "Digital IO Port 1"() -> (w584:u8)
          n342 = global read "CRYMessage Global.vi" "Digital IO Port 2"() -> (w577:u8)
          n343 = property on="serial line state" class="Bool (strict)"("Visible"=w589) -> ()  [unwired: 2 in, 2 out]
          n344 = Not(x=w582) -> (.not. x?=w585:u8)
          n345 = Not(x=w572) -> (.not. x?=w575:u8)
          n346 = And(x=w583, y=w582) -> (x .and. y?=w580:u8)
          n347 = And(x=w585, y=w584) -> (x .and. y?=w581:u8)
          n348 = And(x=w573, y=w572) -> (x .and. y?=w579:u8)
          n349 = And(x=w575, y=w577) -> (x .and. y?=w578:u8)
          n350 = Or(x=w580, y=w581) -> (x .or. y?=w570:u8)
          n351 = Or(x=w579, y=w578) -> (x .or. y?=w562:u8)
          n352 = call "CRYDigital IO H Port Convert.vi"("In Data"=w562) -> ("Out Data"=w561:u8)  [unwired: 10 in]
          n353 = call "CRYMessage Set DigitalIO Ports.vi"("RawPort 2 Pattern"=w562, "Port 2 Pattern"=w561, "Port 1 Pattern"=w570) -> ("Pattern2 Result"=w566:bool, "bInited"=w568:bool, "Pattern1 Result"=w567:bool)  [unwired: 6 in]
          n354 = property on="Write Pattern" class="Clust (strict)"("Visible"=FALSE) -> ()  [unwired: 2 in, 2 out]
          n355 = case shown="True" w568 {
            selector: w568 -> [w591 _]
            tunnel: w567 -> [_ w597]
            tunnel: w566 -> [_ w598]
            tunnel: [w591 w596] -> w565
            frame False {
              n356 = call "CRYGet Error Message.vi"("Error No"=3 ("No"), "Kind"="Messages") -> ("Message"=w595:string, "Window Title"=w594:string)  [unwired: 4 in, 4 out]
              n357 = call "CRYMessage Dialog.vi"("Window Title"=w594, "Message Content"=w595) -> ()  [unwired: 8 in, 2 out]
            }
            frame True {
              n358 = case shown="False" w597 {
                frame False {
                  n359 = call "CRYGet Error Message.vi"("Error No"=4 ("No"), "Kind"="Messages") -> ("Message"=w606:string, "Window Title"=w605:string)  [unwired: 4 in, 4 out]
                  n360 = call "CRYMessage Dialog.vi"("Window Title"=w605, "Message Content"=w606) -> ()  [unwired: 8 in, 2 out]
                }
                frame True {
                }
              }
              n361 = case shown="False" w598 {
                frame False {
                  n362 = call "CRYGet Error Message.vi"("Error No"=5 ("No"), "Kind"="Messages") -> ("Message"=w602:string, "Window Title"=w601:string)  [unwired: 4 in, 4 out]
                  n363 = call "CRYMessage Dialog.vi"("Window Title"=w601, "Message Content"=w602) -> ()  [unwired: 8 in, 2 out]
                }
                frame True {
                }
              }
              n364 = And(x=w597, y=w598) -> (x .and. y?=w596:bool)
            }
          }
          n365 = case shown="..0" w571 {
            tunnel: [TRUE ("Verdict") FALSE ("Verdict")] -> w564
            frame ..0 {
            }
            frame 1.. {
            }
          }
          n366 = And(x=w565, y=w564) -> (x .and. y?=w563:bool)
        }
      }
    }
    frame 2 {
      # "Interface"
      n367 = Greater Than 0?(x=w612) -> (x > 0?=w611:bool)
      n368 = case shown="True" w611 {
        tunnel: w616 -> [_ w640]
        tunnel: w615 -> [_ w626]
        tunnel: [FALSE w625] -> w614
        tunnel: w613 -> [_ w623]
        frame False {
          n369 = call "CRYGet Error Message.vi"("Error No"=1 ("No"), "Kind"="Messages") -> ("Message"=w620:string, "Window Title"=w619:string)  [unwired: 4 in, 4 out]
          n370 = call "CRYMessage Dialog.vi"("Window Title"=w619, "Message Content"=w620) -> ()  [unwired: 8 in, 2 out]
        }
        frame True {
          w622 = FALSE
          n371 = Unbundle By Name(w640) -> ("Flags"=w632:u16, "Pause [ms]"=w633:i32, "Wait?"=w627:bool, "Address"=w636:string, "GPIB term"=w634:i32, "Operation"=w637:i32, "bytes"=w635:i32, "Command Msg"=w639:string, "GPIB func"=w638:u16, "GPIB cmd"=w630:u16, "GPIB rem en"=w631:bool, "RS232 Func"=w629:u16, "Serial Ctrl lines"=w628:u16)
          n372 = case shown="0" w623 {
            tunnel: w639 -> [w653 w782]
            tunnel: w638 -> [_ w793]
            tunnel: w633 -> [w650 w792]
            tunnel: w637 -> [w649 w791]
            tunnel: w636 -> [_ w790]
            tunnel: w635 -> [_ w789]
            tunnel: w634 -> [_ w788]
            tunnel: w632 -> [w654 w787]
            tunnel: [w647 w785] -> w625
            tunnel: w631 -> [_ w784]
            tunnel: w630 -> [_ w783]
            tunnel: w629 -> [w656 _]
            tunnel: w628 -> [w655 _]
            tunnel: w627 -> [w651 w775]
            tunnel: w626 -> [w648 _]
            tunnel: [w645 w780] -> w624
            frame Default {
              # "RS-232 & Others"
              n373 = Equal To 0?(x=w654) -> (x = 0?=w652:bool)
              n374 = case shown="0, Default" w656 {
                tunnel: w655 -> [_ w690 w730]
                tunnel: w652 -> [w664 w688 w733]
                tunnel: w653 -> [w663 w687 _]
                tunnel: w651 -> [w661 w692 w735]
                tunnel: w650 -> [w660 w691 w734]
                tunnel: w649 -> [w662 _ _]
                tunnel: w648 -> [w659 w689 w731]
                tunnel: [w665 w687 _] -> w646
                tunnel: [w658 w688 w732] -> w647
                tunnel: [w657 w686 w729] -> w645
                frame 0, Default {
                  # "Operation tells if it is a read or write"
                  # "write/read message"
                  n375 = Equal To 0?(x=w662) -> (x = 0?=w671:bool)
                  n376 = Or(x=w661, y=w671) -> (x .or. y?=w670:bool)
                  n377 = call "CRYAscii Codes Decode.vi"("String in, with codes"=w663) -> ("String out, decoded"=w666:string)  [unwired: 10 out]
                  n378 = Select(t=w660, s=w670, f=u32 0 ("Timeout (ms)")) -> (s? t:f=w668:u32)
                  n379 = call "CRYSerial Write and Read All.vi"("Read only (F)"=w671, "Timeout (ms)"=w668, "Com port"=w659, "String to write"=w666) -> ("no error"=w657:errorcluster, "Reply received"=w669:string)  [unwired: 6 out]
                  n380 = case shown="False" w671 {
                    tunnel: w666 -> [w677 w682]
                    tunnel: [w675 w683] -> w665
                    tunnel: w669 -> [w673 w681]
                    tunnel: [w672 w678] -> w658
                    tunnel: w664 -> [w672 w680]
                    frame False {
                      n381 = Concatenate Strings("Serial command:\n", w677, "\n\nSerial reply:\n", w673) -> (w675:string)
                    }
                    frame True {
                      n382 = Equal?(x=w681, y=w682) -> (x = y?=w679:bool)
                      n383 = Concatenate Strings("Serial message received:\n", w681) -> (w683:string)
                      n384 = Not Exclusive Or(1:w680, 2:w679) -> (0:w678:bool)
                    }
                  }
                }
                frame 1 {
                  # "set control line"
                  n385 = case shown="True" TRUE {
                    tunnel: w691 -> [_ w704]
                    tunnel: w692 -> [_ w703]
                    tunnel: w689 -> [_ w701]
                    tunnel: w690 -> [_ w695]
                    tunnel: w687 -> [_ _]
                    tunnel: [errorcluster {"status"=FALSE, "code"=0, "source"=""} ("error out") w694] -> w686
                    frame False {
                    }
                    frame True {
                      n386 = Increment(x=w701) -> (x+1=w700:u8)
                      n387 = global read "CRYRef nums global.vi" "VISA serial ports"() -> (w702:T29)
                      n388 = for {
                        tunnel: w702 -> [w727] mode=indexing
                        tunnel: [w726] -> w699 mode=indexing
                        n389 = Unbundle(w727) -> ("COM port (1 = COM1, etc.)"=w726:i32)  [unwired: 1 out]
                      }
                      n390 = Search 1D Array(1D array=w699, element=w700) -> (index of element=w697:i32)  [unwired: 1 out]
                      n391 = Greater Or Equal To 0?(x=w697) -> (x >= 0?=w698:bool)
                      n392 = case shown="True" w698 {
                        tunnel: w702 -> [_ w712]
                        tunnel: w697 -> [_ w711]
                        tunnel: w695 -> [_ w709]
                        tunnel: [w705 w707] -> w694
                        tunnel: errorcluster {"status"=FALSE, "code"=0, "source"=""} ("error out") -> [w705 w706]
                        frame False {
                        }
                        frame True {
                          n393 = Index Array(array=w712, index=w711) -> (element=w710:T30)
                          n394 = Unbundle(w710) -> ("VISA session (for class)"=w708:refnum<visa-resource-name>)  [unwired: 1 out]
                          n395 = case shown="0" w709 {
                            tunnel: w708 -> [w715 w718 w721 w724 _]
                            tunnel: [w713 w716 w719 w722 w725] -> w707
                            tunnel: w706 -> [_ _ _ _ w725]
                            frame 0 {
                              w714 = i16 0 items=["Unknown"=-1, "Unasserted"=0, "Asserted"=1] ("Modem Line Settings:Line DTR State")
                              n396 = property class="Serial Instr"(reference=w715, "Serial Settings:Modem Line Settings:Line DTR State"=w714) -> (error out=w713:errorcluster)  [unwired: 1 in, 1 out]
                            }
                            frame 1 {
                              w717 = i16 1 items=["Unknown"=-1, "Unasserted"=0, "Asserted"=1] ("Modem Line Settings:Line DTR State")
                              n397 = property class="Serial Instr"(reference=w718, "Serial Settings:Modem Line Settings:Line DTR State"=w717) -> (error out=w716:errorcluster)  [unwired: 1 in, 1 out]
                            }
                            frame 2 {
                              w720 = i16 0 items=["Unknown"=-1, "Unasserted"=0, "Asserted"=1] ("Modem Line Settings:Line DTR State")
                              n398 = property class="Serial Instr"(reference=w721, "Serial Settings:Modem Line Settings:Line RTS State"=w720) -> (error out=w719:errorcluster)  [unwired: 1 in, 1 out]
                            }
                            frame 3 {
                              w723 = i16 1 items=["Unknown"=-1, "Unasserted"=0, "Asserted"=1] ("Modem Line Settings:Line DTR State")
                              n399 = property class="Serial Instr"(reference=w724, "Serial Settings:Modem Line Settings:Line RTS State"=w723) -> (error out=w722:errorcluster)  [unwired: 1 in, 1 out]
                            }
                            frame Default {
                            }
                          }
                        }
                      }
                      n400 = case shown="True" w703 {
                        tunnel: w704 -> [_ w728]
                        tunnel: w694 -> [_ _]
                        frame False {
                        }
                        frame True {
                          n401 = Wait (ms)(milliseconds to wait=w728) -> ()  [unwired: 1 out]
                        }
                      }
                    }
                  }
                }
                frame 2 {
                  w744 = i16 1 items=["Unknown"=-1, "Unasserted"=0, "Asserted"=1] ("Modem Line Settings:Line DTR State")
                  # "read control line"
                  n402 = global read "CRYRef nums global.vi" "VISA serial ports"() -> (w736:T29)
                  n403 = case shown="True" w735 {
                    tunnel: [u32 0 ("millisecond timer value") w774] -> w742
                    tunnel: w734 -> [_ w773]
                    frame False {
                    }
                    frame True {
                      n404 = Wait (ms)(milliseconds to wait=w773) -> (millisecond timer value=w774:u32)
                    }
                  }
                  n405 = Increment(x=w731) -> (x+1=w737:u8)
                  n406 = for {
                    tunnel: w736 -> [w771] mode=indexing
                    tunnel: [w770] -> w738 mode=indexing
                    n407 = Unbundle(w771) -> ("COM port (1 = COM1, etc.)"=w770:i32)  [unwired: 1 out]
                  }
                  n408 = Search 1D Array(1D array=w738, element=w737) -> (index of element=w740:i32)  [unwired: 1 out]
                  n409 = Greater Or Equal To 0?(x=w740) -> (x >= 0?=w739:bool)
                  n410 = case shown="True" w739 {
                    tunnel: w736 -> [_ w755]
                    tunnel: w740 -> [_ w754]
                    tunnel: w730 -> [_ w752]
                    tunnel: [w747 w750] -> w729
                    tunnel: errorcluster {"status"=FALSE, "code"=0, "source"=""} ("error out") -> [w747 w749]
                    tunnel: w742 -> [_ _]
                    tunnel: [w746 w748] -> w743
                    frame False {
                      w746 = i16 0 items=["Unknown"=-1, "Unasserted"=0, "Asserted"=1] ("Modem Line Settings:Line DTR State")
                    }
                    frame True {
                      n411 = Index Array(array=w755, index=w754) -> (element=w753:T30)
                      n412 = Unbundle(w753) -> ("VISA session (for class)"=w751:refnum<visa-resource-name>)  [unwired: 1 out]
                      n413 = case shown="0" w752 {
                        tunnel: w751 -> [w758 w761 w764 w767 _]
                        tunnel: [w757 w760 w763 w766 w769] -> w750
                        tunnel: w749 -> [_ _ _ _ w769]
                        tunnel: [w756 w759 w762 w765 w768] -> w748
                        frame 0 {
                          n414 = property class="Serial Instr"(reference=w758) -> (error out=w757:errorcluster, "Serial Settings:Modem Line Settings:Line DCD State"=w756:i16)  [unwired: 1 in, 1 out]
                        }
                        frame 1 {
                          n415 = property class="Serial Instr"(reference=w761) -> (error out=w760:errorcluster, "Serial Settings:Modem Line Settings:Line DSR State"=w759:i16)  [unwired: 1 in, 1 out]
                        }
                        frame 2 {
                          n416 = property class="Serial Instr"(reference=w764) -> (error out=w763:errorcluster, "Serial Settings:Modem Line Settings:Line CTS State"=w762:i16)  [unwired: 1 in, 1 out]
                        }
                        frame 3 {
                          n417 = property class="Serial Instr"(reference=w767) -> (error out=w766:errorcluster, "Serial Settings:Modem Line Settings:Line RI State"=w765:i16)  [unwired: 1 in, 1 out]
                        }
                        frame Default {
                          w768 = i16 0 items=["Unknown"=-1, "Unasserted"=0, "Asserted"=1] ("Modem Line Settings:Line DTR State")
                        }
                      }
                    }
                  }
                  n418 = Equal?(x=w743, y=w744) -> (x = y?=w745:bool)
                  "serial line state" <- w745
                  n419 = Not Exclusive Or(1:w745, 2:w733) -> (0:w732:bool)
                }
              }
              n420 = property on="Command" class="Str"("Value"=w646) -> ()  [unwired: 2 in, 2 out]
            }
            frame 0 {
              # "IEEE-488"
              n421 = Equal To 0?(x=w787) -> (x = 0?=w786:bool)
              n422 = case shown="1" w793 {
                tunnel: w775 -> [w812 _ _ _]
                tunnel: w792 -> [w811 _ _ w898]
                tunnel: w791 -> [w809 _ _ _]
                tunnel: w790 -> [w807 w835 w885 w903]
                tunnel: w789 -> [w806 _ _ _]
                tunnel: w788 -> [w800 _ _ _]
                tunnel: [w805 w838 w891 w902] -> w780
                tunnel: [w804 w839 w889 w899] -> w781
                tunnel: w782 -> [w799 _ _ _]
                tunnel: w786 -> [w803 w841 w890 w901]
                tunnel: [w801 w840 w888 w900] -> w785
                tunnel: w784 -> [_ w845 _ _]
                tunnel: w783 -> [_ w843 _ _]
                tunnel: [w797 w835 w885 w896] -> w779
                tunnel: [w796 w834 w884 bool[] [] ("status")] -> w778
                tunnel: [w794 TRUE TRUE FALSE ("Dialog?(F)")] -> w777
                tunnel: [w795 w832 "Serial Poll" w896] -> w776
                frame 0, Default {
                  # "write/read message"
                  n423 = call "CRYAscii Codes Decode.vi"("String in, with codes"=w799) -> ("String out, decoded"=w798:string)  [unwired: 10 out]
                  n424 = Select(t=w811, s=w812, f=0) -> (s? t:f=w808:i32)
                  n425 = case shown="1" w809 {
                    tunnel: w808 -> [w823 _]
                    tunnel: w807 -> [w816 w827]
                    tunnel: w806 -> [w822 _]
                    tunnel: [w820 w829] -> w805
                    tunnel: [w818 w831] -> w804
                    tunnel: w798 -> [w819 w831]
                    tunnel: [w817 w828] -> w802
                    tunnel: w800 -> [_ w830]
                    tunnel: [w816 w827] -> w797
                    tunnel: [w815 w826] -> w796
                    tunnel: ["GPIB Read" "GPIB Write"] -> w795
                    tunnel: [TRUE ("Dialog?(F)") TRUE ("Dialog?(F)")] -> w794
                    frame 0, Default {
                      # "Read"
                      n426 = GPIB Read(0:w816, 1:w822, 2:i16 0 ("mode (0)"), 4:w823) -> (5:w818:string, 6:w815:bool[], 7:w820:errorcluster)  [unwired: 1 in]
                      n427 = Equal?(x=w818, y=w819) -> (x = y?=w817:bool)
                    }
                    frame 1 {
                      # "Write"
                      n428 = GPIB Write(0:w827, 1:w831, 2:w830) -> (5:w826:bool[], 6:w829:errorcluster)  [unwired: 1 in, 1 out]
                      n429 = And Array Elements(Boolean array=w826) -> (logical AND=w828:bool)
                    }
                  }
                  n430 = Not Exclusive Or(1:w802, 2:w803) -> (0:w801:bool)
                }
                frame 1 {
                  # "interface message"
                  n431 = Select(t="sre 1", s=w845, f="sre 0") -> (s? t:f=w837:string)
                  n432 = GPIB Misc(0:w837) -> (4:w836:errorcluster)  [unwired: 1 in, 2 out]
                  n433 = case shown="1" w843 {
                    tunnel: [w848 w857 w863 w871 w876 w883] -> w834
                    tunnel: [w849 w859 w862 w870 w875 w882] -> w838
                    tunnel: w835 -> [_ w858 w864 w867 _ _]
                    tunnel: ["Device Clear" "Selected Device Clear" "Group Execute Trigger" "Go to Local" "Local Lockout" "Unlisten"] -> w832
                    tunnel: [w850 "" "" w868 w872 w880] -> w839
                    tunnel: w836 -> [w847 _ _ _ _ _]
                    frame 0, Default {
                      # "device clear"
                      n434 = Concatenate Strings("cmd ", "DCL") -> (w853:string)
                      n435 = GPIB Misc(0:w853, 1:w847) -> (2:w850:string, 3:w848:bool[], 4:w849:errorcluster)
                    }
                    frame 1 {
                      # "selected dev clr"
                      n436 = GPIB Clear(3:w858) -> (0:w859:errorcluster, 1:w857:bool[])  [unwired: 1 in]
                    }
                    frame 2 {
                      # "group exec trigger"
                      n437 = GPIB Trigger(3:w864) -> (0:w862:errorcluster, 1:w863:bool[])  [unwired: 1 in]
                    }
                    frame 3 {
                      # "go to local"
                      n438 = Concatenate Strings("loc ", w867) -> (w865:string)
                      n439 = GPIB Misc(0:w865) -> (2:w868:string, 3:w871:bool[], 4:w870:errorcluster)  [unwired: 1 in]
                    }
                    frame 4 {
                      # "local lockout"
                      n440 = GPIB Misc(0:"llo" ("command string")) -> (2:w872:string, 3:w876:bool[], 4:w875:errorcluster)  [unwired: 1 in]
                    }
                    frame 5 {
                      # "unlisten"
                      n441 = Concatenate Strings("cmd ", "UNL") -> (w878:string)
                      n442 = GPIB Misc(0:w878) -> (2:w880:string, 3:w883:bool[], 4:w882:errorcluster)  [unwired: 1 in]
                    }
                  }
                  n443 = And Array Elements(Boolean array=w834) -> (logical AND=w842:bool)
                  n444 = Not Exclusive Or(1:w842, 2:w841) -> (0:w840:bool)
                }
                frame 2 {
                  # "serial poll"
                  n445 = GPIB Serial Poll(0:w885) -> (2:w893:i16, 3:w884:bool[], 4:w891:errorcluster)  [unwired: 1 in]
                  n446 = And Array Elements(Boolean array=w884) -> (logical AND=w894:bool)
                  n447 = Format Into String(format string="%016b" ("Format String"), w893) -> (resulting string=w889:string)  [unwired: 2 in, 1 out]
                  n448 = Not Exclusive Or(1:w894, 2:w890) -> (0:w888:bool)
                }
                frame 3 {
                  w896 = "" ("Address")
                  # "wait for service request"
                  n449 = Wait for GPIB RQS(3:w898, 4:w903) -> (0:w902:errorcluster, 1:w905:i16)  [unwired: 1 in]
                  n450 = Not Equal?(x=w905, y=i16 -1 ("Input 1")) -> (x != y?=w907:bool)
                  n451 = Format Into String(format string="%016b" ("Format String"), w905) -> (resulting string=w899:string)  [unwired: 2 in, 1 out]
                  n452 = Not Exclusive Or(1:w907, 2:w901) -> (0:w900:bool)
                }
              }
              n453 = call "CRYGPIB Error Report.vi"("Function"=w776, "Dialog?(F)"=w777, "Status"=w778, "Address String"=w779) -> ()  [unwired: 2 out]
              n454 = property on="Command" class="Str"("Value"=w781) -> ()  [unwired: 2 in, 2 out]
            }
          }
          n455 = property on="OK" class="Bool (strict)"("Visible"=w622) -> ()  [unwired: 2 in, 2 out]
          n456 = property on="pattern" class="Str"("Visible"=w622) -> ()  [unwired: 2 in, 2 out]
          n457 = property on="Numeric" class="DigNum (strict)"("Visible"=w622) -> ()  [unwired: 2 in, 2 out]
          n458 = property on="Pattern read" class="Clust (strict)"("Visible"=w622) -> ()  [unwired: 2 in, 2 out]
          n459 = property on="unit" class="Str"("Visible"=w622) -> ()  [unwired: 2 in, 2 out]
          n460 = property on="Yes" class="Bool (strict)"("Visible"=w622) -> ()  [unwired: 2 in, 2 out]
          n461 = property on="Write Pattern" class="Clust (strict)"("Visible"=w622) -> ()  [unwired: 2 in, 2 out]
          n462 = property on="No" class="Bool (strict)"("Visible"=w622) -> ()  [unwired: 2 in, 2 out]
          n463 = property on="Time" class="Slide (strict)"("Visible"=w622) -> ()  [unwired: 2 in, 2 out]
          n464 = property on="serial line state" class="Bool (strict)"("Visible"=w622) -> ()  [unwired: 2 in, 2 out]
          n465 = case shown="Error" w624 {
            selector: w624 -> [_ w644]
            frame No Error {
            }
            frame Error {
              n466 = Unbundle By Name(w644) -> ("source"=w641:string)
              n467 = call "CRYGet Error Message.vi"() -> ("Window Title"=w642:string)  [unwired: 6 in, 5 out]
              n468 = call "CRYMessage Dialog.vi"("Window Title"=w642, "YesNoCancel"=T17."OK", "Message Content"=w641) -> ()  [unwired: 7 in, 2 out]
            }
          }
        }
      }
    }
  }
  n469 = Index Array(array=w11, index=1) -> (element=w13:bool)
  n470 = global read "CRYProject Run Control Global.vi" "RunState"() -> (w9:bool)
  n471 = Select(t="Overwrite" ("Y unit"), s=w13, f="Repeat") -> (s? t:f=w14:string)
  n472 = flat-sequence {
    tunnel: w24 -> [w919]
    tunnel: w25 -> [w911]
    tunnel: "Step name" -> [w920]
    tunnel: [w920] -> w17
    tunnel: [w911] -> w16
    tunnel: [w919] -> w15
    tunnel: w14 -> [w918]
    tunnel: w13 -> [w912]
    tunnel: w12 -> [w917]
    tunnel: w8 -> [w916]
    tunnel: w7 -> [w915]
    tunnel: w4 -> [w914]
    tunnel: w3 -> [w913]
    tunnel: w17 -> [w932]
    tunnel: w16 -> [w931]
    tunnel: w15 -> [w929]
    frame #0 {
      n473 = case shown="False" w912 {
        tunnel: w914 -> [w926 w928]
        tunnel: w913 -> [w925 w927]
        tunnel: [w924 w927] -> w910
        tunnel: [w923 w928] -> w909
        tunnel: w917 -> [w922 _]
        tunnel: w915 -> [w921 _]
        frame False {
          n474 = call "CRYPrefix Curve Name.vi"("Type In"=w921, "Values In"=w926, "Results In"=w925, "Repeat State Array In"=w922) -> ("Values Out"=w923:T31, "Results Out"=w924:T4)  [unwired: 8 in, 2 out]
        }
        frame True {
        }
      }
      n475 = call "CRYInsert Socket.vi"("sOption2"=w918, "Step No."=w911, "sOption1"=w916, "Results"=w910, "Values"=w909) -> ("Inserted Names Out"=→"Inserted Names Out":string[])  [unwired: 6 in]
    }
    frame #1 {
      n476 = call "CRYUnflatten Results.vi"() -> ("Result"=w930:T5)  [unwired: 9 in, 2 out]
      n477 = Bundle By Name(cluster=w930, "Name"=w932, "Verdict"=w929, "Step No."=w931) -> (w934:T5)
      n478 = Build Array(w934) -> (→"Results out":T5[])
    }
  }
  n479 = case shown="True" w9 {
    tunnel: ["Apply" ("sOption1") "Run" ("Type In")] -> w8
    tunnel: ["APPLY_CURVE" ("Type In") "RUN_CURVE" ("Type In")] -> w7
    frame False {
    }
    frame True {
    }
  }
